vi "sub_SDR_tx_GenerateFramePayload.vi"(6 "Init?":bool, 10 "Packets":string[](array[string]), 11 "Payload Length":i32) -> (0 "Buffer Length":i32, 2 "Payload String":string, 3 "Link occupation [%]":dbl)   [LabVIEW 2012]
uses:
  <vilib>/gmath/statdist.llb/Uniform Random.vi
  <vilib>/gmath/NI_Gmath.lvlib
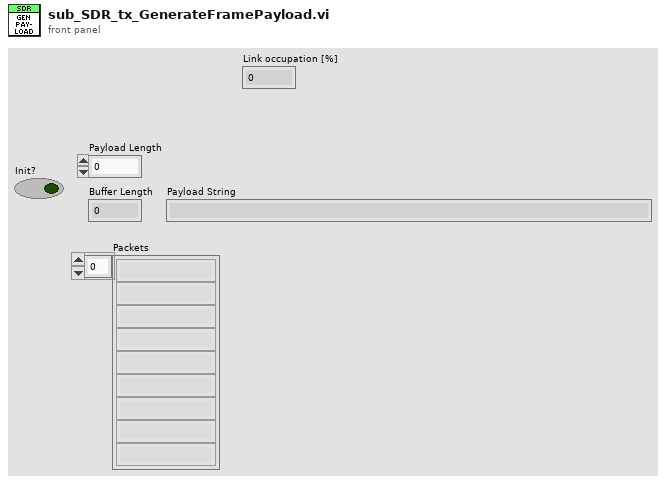
[diagram p1: front panel]
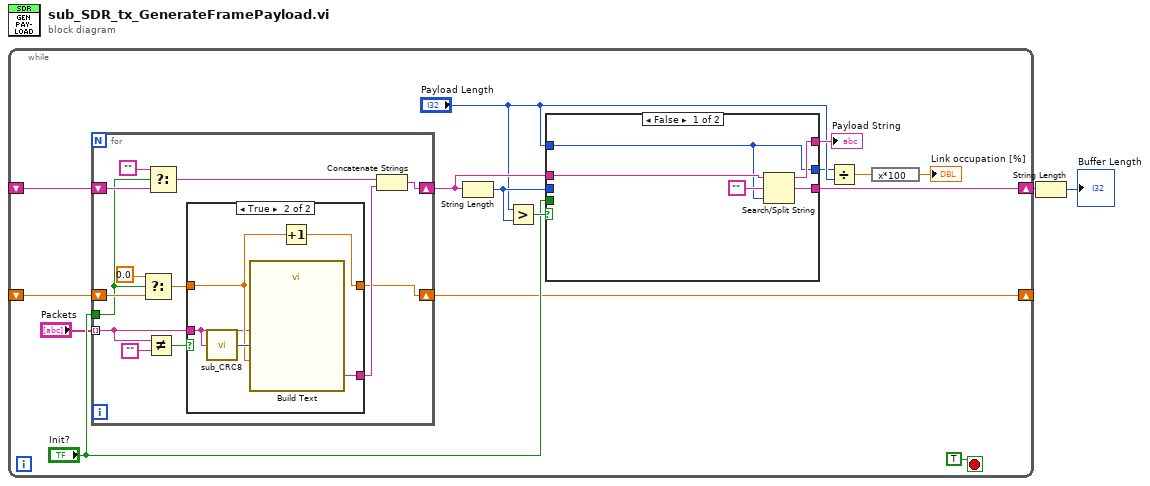
[diagram p0: block diagram]
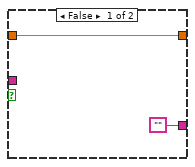
[diagram p2: hidden frame]
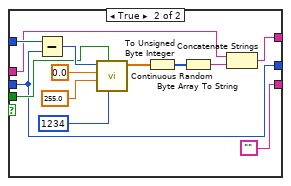
[diagram p3: hidden frame]
diagram:
  n1 = while {
    shift-right: [w13] -> w2
    shift-left: _ -> [w12]
    shift-right: [w8] -> _
    shift-left: _ -> [w10]
    stop <- TRUE stop-if-true
    n2 = for {
      tunnel: "Init?" -> [w21]
      shift-right: [w25] -> w15
      shift-left: w12 -> [w24]
      tunnel: "Packets" -> [w18] mode=indexing
      shift-right: [w19] -> w8
      shift-left: w10 -> [w22]
      n3 = Select(t=0.0, s=w21, f=w22) -> (s? t:f=w23:dbl)
      n4 = Not Equal?(x=w18, y="") -> (x != y?=w30:bool)
      n5 = Select(t="", s=w21, f=w24) -> (s? t:f=w26:string)
      n6 = case shown="True" w30 {
        tunnel: ["" w36] -> w28
        tunnel: w23 -> [w31 w35]
        tunnel: [w31 w34] -> w19
        tunnel: w18 -> [_ w33]
        frame False {
        }
        frame True {
          n7 = call "sub_CRC8.vi"("message"=w33) -> ("CRC8"=w37:u8)  [unwired: 4 in]
          n8 = call "Build Text"("PKT#"=w35, "CRC"=w37, "Packet"=w33) -> ("Result"=w36:string)  [unwired: 11 in, 1 out]
          n9 = Increment(x=w35) -> (x+1=w34:dbl)
        }
      }
      n10 = Concatenate Strings(w26, w28) -> (w25:string)
    }
    n11 = String Length(string=w15) -> (length=w14:i32)
    n12 = Greater?(x="Payload Length", y=w14) -> (0:w16:bool)
    n13 = case shown="False" w16 {
      tunnel: [w41 w53] -> w11
      tunnel: "Payload Length" -> [w38 w47]
      tunnel: "Init?" -> [_ w46]
      tunnel: w15 -> [w42 w45]
      tunnel: w14 -> [_ w43]
      tunnel: [w40 ""] -> w13
      tunnel: [w38 w43] -> w5
      frame False {
        n14 = Search/Split String(string=w42, search string/char (-)="", offset (0)=w38) -> (substring before match=w41:string, match + rest of string=w40:string)  [unwired: 1 out]
      }
      frame True {
        n15 = Subtract(x=w47, y=w43) -> (x-y=w49:i32)
        n16 = call-poly <vilib>:"Continuous Random.vi"("seed"=1234, "reset"=w46, "xmax"=255.0, "xmin"=0.0, "samples"=w49) -> ("uniform random data"=w54:dbl[])  [unwired: 5 in, 1 out]
        n17 = To Unsigned Byte Integer(number=w54) -> (unsigned 8bit integer=w55:u8[])
        n18 = Byte Array To String(unsigned byte array=w55) -> (string=w48:string)
        n19 = Concatenate Strings(w45, w48) -> (w53:string)
      }
    }
    "Payload String" <- w11
    n20 = Divide(x=w5, y="Payload Length") -> (x/y=w4:dbl)
    n21 = expression code="x*100"(w4) -> (→"Link occupation [%]":dbl)
  }
  n22 = String Length(string=w2) -> (length=→"Buffer Length":i32)
